vi "Is Message Well Known Type.vi"(1 "repeated":bool, 2 "message name":string) -> (0 "well known type":T1)   [LabVIEW 2019, in "grpc-lvsupport.lvlib"]
uses:
  grpc-lvsupport.lvlib
  Well Known Types.ctl
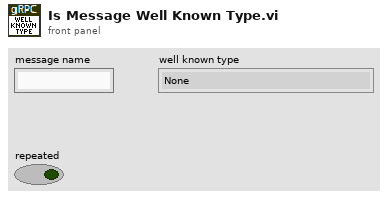
[diagram p1: front panel]
types:
  T1 = typedef "grpc-lvsupport.lvlib/Well Known Types.ctl" = enum32{"None", "Double2DArray", "String2DArray"}
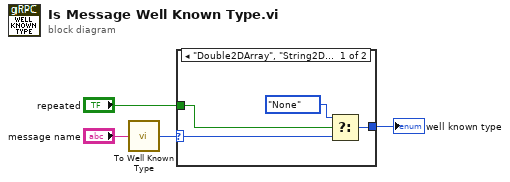
[diagram p0: block diagram]
diagram:
  n1 = call "To Well Known Type.vi"("message name"="message name") -> ("well known type"=w2:T1)
  n2 = case shown="\"Double2DArray\", \"String2DArray\"" w2 {
    selector: w2 -> [w7 w9]
    tunnel: "repeated" -> [w8 _]
    tunnel: [w5 w9] -> w1
    frame "Double2DArray", "String2DArray" {
      n3 = Select(t=Well_Known_Types."None", s=w8, f=w7) -> (s? t:f=w5:T1)
    }
    frame "None" {
    }
  }
  "well known type" <- w1
